vi "SSL_Connect_With_Keys.vi"(8 "error in (no error)":errorcluster, 9 "cert path":T1={"client cert file"=path "", "CA file"=path "", "client key file"=path ""}, 10 "SSL_Connection":T2, 11 "login":T3={"server IP"="", "server port"=0, "local port (0 = auto)"=0, "timeout ms (1000)"=1000}) -> (0 "error out":errorcluster, 2 "SSL_Connection":T2)   [LabVIEW 2015, in "AWS_IoT.lvlib"]
uses:
  AWS_IoT.lvlib
  Controls/SSL_login.ctl
  Controls/SSL_Connection.ctl
  Controls/certs.ctl
  <vilib>/httpClient/LabVIEWHTTPClient.lvlib
panel:
  out "Numeric":i32
  out "return type 2":i32
  out "cert error":bool
  out "return type":i32
  out "connection status":i32
  out "retCode":i32
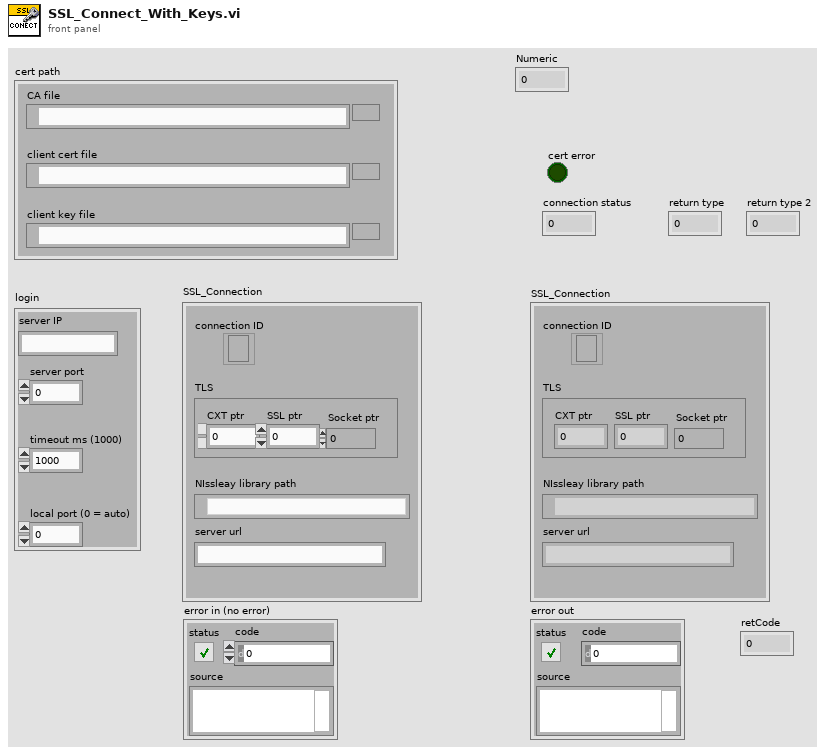
[diagram p1: front panel]
types:
  T1 = typedef "AWS_IoT.lvlib/certs.ctl" = cluster{"client cert file":path, "CA file":path, "client key file":path}
  T2 = typedef "AWS_IoT.lvlib/SSL_Connection.ctl" = cluster{"connection ID":refnum<k5>, "TLS":cluster{"CXT ptr":i32, "SSL ptr":i32, "Socket ptr":u64}, "NIssleay library path":path, "server url":string}
  T3 = typedef "AWS_IoT.lvlib/SSL_login.ctl" = cluster{"server IP":string, "server port":u16, "local port (0 = auto)":u16, "timeout ms (1000)":i32}
  T4 = typedef "LabVIEWHTTPClient.lvlib/ClientHandle.ctl" = refnum<k1>
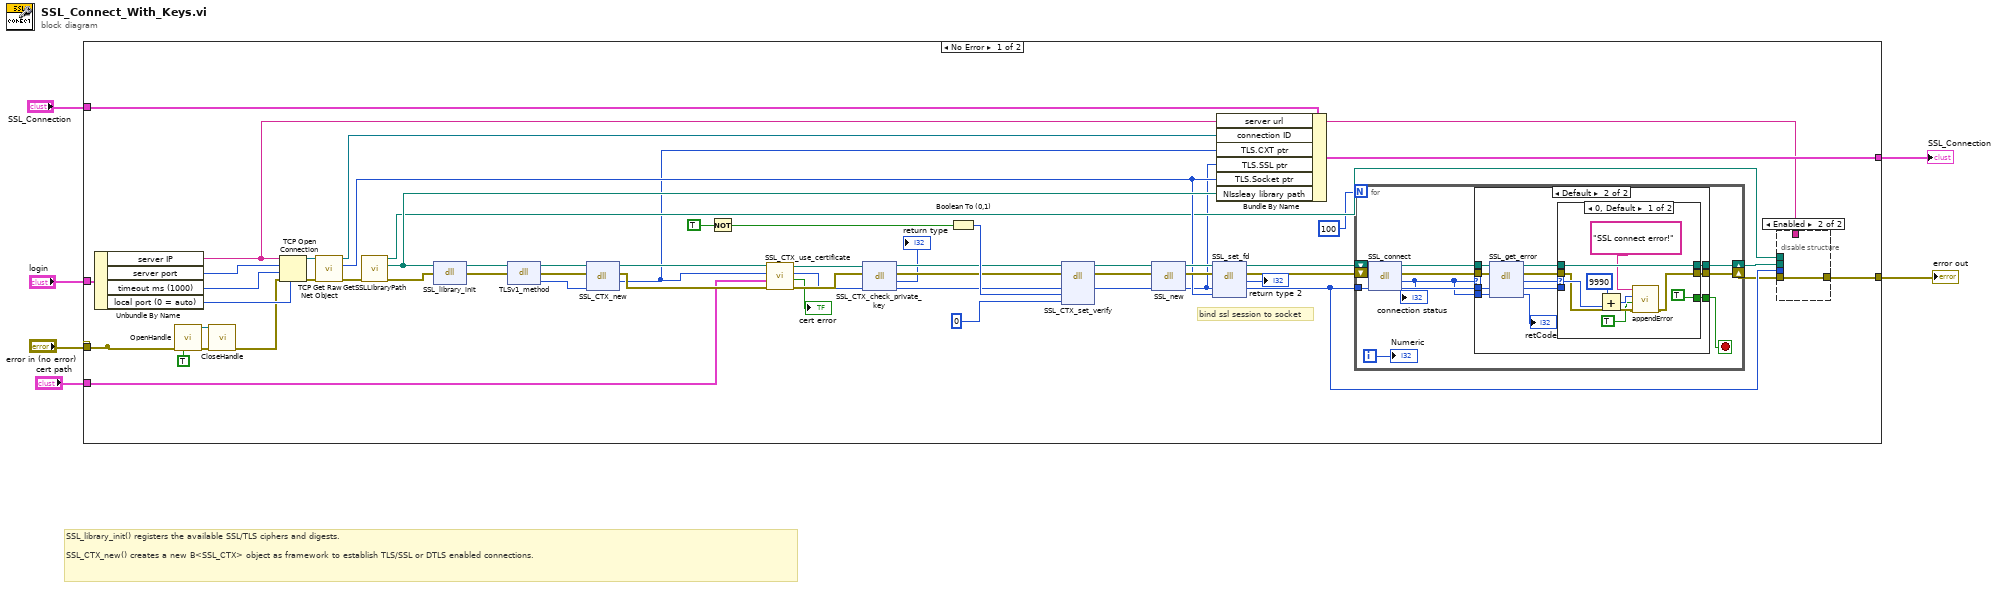
[diagram p0: block diagram]
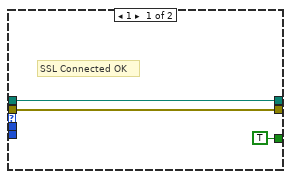
[diagram p2: hidden frame]
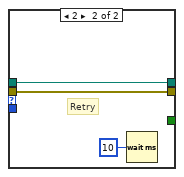
[diagram p3: hidden frame]
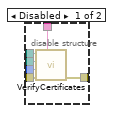
[diagram p4: hidden frame]
diagram:
  # "SSL_library_init() registers the available SSL/TLS ciphers and digests.\n\nSSL_CTX_new() creates a new B<SSL_CTX> object as framework to establish TLS/SSL or DTLS enabled connections."
  n1 = case shown="No Error" "error in (no error)" {
    selector: "error in (no error)" -> [w32 w107]
    tunnel: "login" -> [w56 _]
    tunnel: "SSL_Connection" -> [w55 w108]
    tunnel: [w35 w108] -> w4
    tunnel: [w32 _] -> _
    tunnel: [w25 w107] -> w3
    tunnel: "cert path" -> [w13 _]
    frame No Error {
      # "bind ssl session to socket"
      n2 = Unbundle By Name(w56) -> ("server IP"=w26:string, "server port"=w59:u16, "timeout ms (1000)"=w58:i32, "local port (0 = auto)"=w57:u16)
      n3 = call <vilib>:"OpenHandle.vi"("error in (no error)"=w32, "verify server(true)"=TRUE) -> ("client handle out"=w34:T4, "error out"=w33:errorcluster)  [unwired: 12 in]
      n4 = call <vilib>:"CloseHandle.vi"("client handle"=w34, "error in (no error)"=w33) -> ("error out"=w31:errorcluster)  [unwired: 13 in]
      n5 = TCP Open Connection(address=w26, remote port or service name=w59, timeout ms (60000)=w58, local port=w57, error in (no error)=w31) -> (connection ID=w61:refnum<k5>, error out=w60:errorcluster)
      n6 = call <vilib>:"TCP Get Raw Net Object.vi"("error in (no error)"=w60, "connection ID"=w61) -> ("error out"=w42:errorcluster, "raw net object"=w39:u64, "connection ID out"=w54:refnum<k5>)  [unwired: 7 in]
      n7 = call "GetSSLLibraryPath.vi"("error in (no error)"=w42) -> ("error out"=w40:errorcluster, "NIssleay library path"=w41:path, "NIlibeay library pat"=w22:path)  [unwired: 7 in, 1 out]
      n8 = dll-call lib="NIssleay32.*" fn="SSL_library_init"(path in=w41, error in=w40) -> (path out=w48:path, error out=w43:errorcluster)  [unwired: 2 in]
      n9 = dll-call lib="NIssleay32.*" fn="TLSv1_method"(path in=w48, error in=w43) -> (path out=w49:path, error out=w44:errorcluster, "return type"=w45:i32)  [unwired: 1 in]
      n10 = dll-call lib="NIssleay32.*" fn="SSL_CTX_new"(path in=w49, error in=w44, "ClientMethod"=w45) -> (path out=w17:path, error out=w15:errorcluster, "return type"=w14:i32)  [unwired: 2 in]
      n11 = Not(x=TRUE) -> (.not. x?=w38:bool)
      n12 = call "SSL_CTX_use_certificate.vi"("error in (no error)"=w15, "cert path"=w13, "CTX"=w14, "path in"=w17) -> ("error out"=w12:errorcluster, "cert error"=→"cert error":bool, "CTX"=w11:i32, "path out"=w16:path)  [unwired: 4 in]
      n13 = dll-call lib="NIssleay32.*" fn="SSL_CTX_check_private_key"(path in=w16, error in=w12, "CTX"=w11) -> (path out=w21:path, error out=w20:errorcluster, "return type"=→"return type":i32, "CTX"=w19:i32)  [unwired: 1 in]
      n14 = Boolean To (0,1)(Boolean=w38) -> (0, 1=w36:i16)
      n15 = dll-call lib="NIssleay32.*" fn="SSL_CTX_set_verify"(path in=w21, error in=w20, "CTX"=w19, "mode"=w36, "verify_callback"=0) -> (path out=w50:path, error out=w51:errorcluster, "CTX"=w52:i32)  [unwired: 4 in]
      n16 = dll-call lib="NIssleay32.*" fn="SSL_new"(path in=w50, error in=w51, "Context"=w52) -> (path out=w46:path, error out=w47:errorcluster, "Context"=w8:i32)  [unwired: 2 in]
      n17 = dll-call lib="NIssleay32.*" fn="SSL_set_fd"(path in=w46, error in=w47, "SSL"=w8, "Socket"=w39) -> (path out=w29:path, error out=w28:errorcluster, "return type"=→"return type 2":i32, "SSL"=w24:i32)  [unwired: 2 in]
      n18 = Bundle By Name(cluster=w55, "server url"=w26, "connection ID"=w54, "TLS.CXT ptr"=w14, "TLS.SSL ptr"=w8, "TLS.Socket ptr"=w39, "NIssleay library path"=w41) -> (w35:T2)
      n19 = for {
        N: 100 -> [_]
        tunnel: w24 -> [w69]
        shift-right: [w70] -> w27
        shift-left: w29 -> [w72]
        shift-right: [w68] -> w23
        shift-left: w28 -> [w71]
        i -> [w63]
        stop <- w62 stop-if-true
        n20 = dll-call lib="NIssleay32.*" fn="SSL_connect"(path in=w72, error in=w71, "SSL"=w69) -> (path out=w67:path, error out=w66:errorcluster, "return type"=w64:i32, "SSL"=w65:i32)  [unwired: 1 in]
        "connection status" <- w64
        n21 = case shown="Default" w64 {
          tunnel: w64 -> [_ w87]
          tunnel: w67 -> [w75 w86]
          tunnel: w66 -> [w74 w85]
          tunnel: [w74 w81] -> w68
          tunnel: [TRUE w79] -> w62
          tunnel: w65 -> [_ w78]
          tunnel: [w75 w82] -> w70
          frame 1 {
            # "SSL Connected OK"
          }
          frame Default {
            n22 = dll-call lib="NIssleay32.*" fn="SSL_get_error"(path in=w86, error in=w85, "SSL"=w78, "retCode"=w87) -> (path out=w83:path, error out=w84:errorcluster, "return type"=w80:i32, "SSL"=w77:i32, "retCode"=→"retCode":i32)  [unwired: 1 in]
            n23 = case shown="0, Default" w80 {
              selector: w80 -> [w94 _]
              tunnel: w84 -> [w90 w97]
              tunnel: w83 -> [w96 w98]
              tunnel: [w96 w98] -> w82
              tunnel: [w91 w97] -> w81
              tunnel: [TRUE _] -> w79
              tunnel: w77 -> [_ _]
              frame 0, Default {
                n24 = Add(x=9990, y=w94) -> (x+y=w92:i32)
                n25 = call "appendError.vi"("error in (no error)"=w90, "Boolean"=TRUE, "code"=w92, "String"="SSL connect error!" ("error message (\"\")")) -> ("error out"=w91:errorcluster)  [unwired: 7 in]
              }
              frame 2 {
                # "Retry"
                n26 = Wait (ms)(milliseconds to wait=u32 10) -> ()  [unwired: 1 out]
              }
            }
          }
        }
        "Numeric" <- w63
      }
      n27 = disable-structure shown="Enabled" {
        disable-tunnel: w27 -> [w105 _]
        disable-tunnel: w26 -> [w104 _]
        disable-tunnel: [w103 w106] -> w25
        disable-tunnel: w24 -> [w102 _]
        disable-tunnel: w23 -> [w101 w106]
        disable-tunnel: w22 -> [w100 _]
        frame Disabled {
          n28 = call "VerifyCertificates.vi"("server url"=w104, "error in (no error)"=w101, "SSL ref"=w102, "NIssleay path"=w105, "NIlibeay path"=w100) -> ("error out"=w103:errorcluster)  [unwired: 6 in]
        }
        frame Enabled {
        }
      }
    }
    frame Error {
    }
  }
  "SSL_Connection" <- w4
  "error out" <- w3
